vi "Enum to String.vi"(11 "Command":variant) -> (2 "Commands []":string[](array[string]), 3 "Command":string)   [LabVIEW 2019, in "Instrument.lvclass"]
uses:
  Instrument.lvclass
  <vilib>/Utility/Data Type/NI_Data Type.lvlib
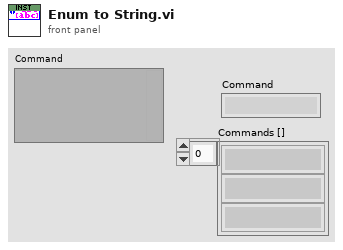
[diagram p1: front panel]
types:
  T1 = typedef "NI_Data Type.lvlib/Data Type.ctl" = enum8{"Invalid Type", "Void", "I8", "I16", "I32", "I64", "U8", "U16", "U32", "U64", "Single Float", "Double Float", "Extended Float", "Single Complex", "Double Complex", "Extended Complex", "Enum U8", "Enum U16", "Enum U32", "Enum U64", "Single Float With Unit", "Double Float With Unit", "Extended Float With Unit", "Single Complex with Unit", "Double Complex with Unit", "Extended Complex with Unit", "Boolean", "String", "Path", "Picture", "Tag", "Array", "Cluster", "Variant", "LV Variant", "Waveform", "Timestamp", "Digital Waveform", "Digital Data", "ExpressData", "Refnum", "External Data", "VI", "Poly VI", "LabVIEW Class Instance", "Fixed Point", "Set Collection", "Map Collection"}
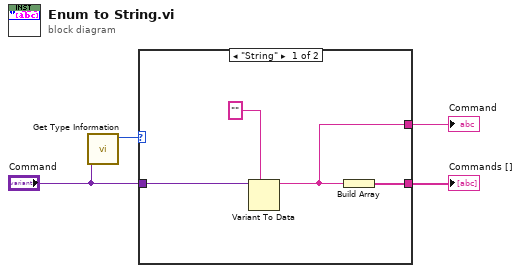
[diagram p0: block diagram]
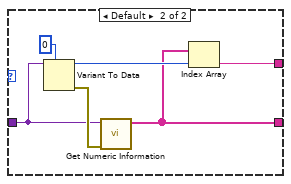
[diagram p2: hidden frame]
diagram:
  n1 = call <vilib>:"Get Type Information.vi"("variant"="Command") -> ("type"=w1:T1)  [unwired: 6 in, 4 out]
  n2 = case shown="\"String\"" w1 {
    tunnel: [w6 w12] -> w4
    tunnel: [w5 w11] -> w3
    tunnel: "Command" -> [w7 w9]
    frame "String" {
      n3 = Variant To Data(type="", Variant=w7) -> (data=w6:string)  [unwired: 1 in, 1 out]
      n4 = Build Array(w6) -> (w5:string[])
    }
    frame Default {
      n5 = Variant To Data(type=0, Variant=w9) -> (data=w13:i32, error out=w10:errorcluster)  [unwired: 1 in]
      n6 = call <vilib>:"Get Numeric Information.vi"("error in (no error)"=w10, "variant"=w9) -> ("enum names"=w11:string[])  [unwired: 6 in, 3 out]
      n7 = Index Array(array=w11, index=w13) -> (element=w12:string)
    }
  }
  "Commands []" <- w3
  "Command" <- w4
